vi "2nd_Order_ODE.vi"(2 "data":T1, 3 "t":dbl, 4 "x":dbl[](array[numeric])) -> (0 "error out":errorcluster, 1 "f(x,t)":dbl[](array[numeric]))   [LabVIEW 2012]
doc: "This template is the starting point for creating a function that is the right-hand-side of an ordinary differential equaltion to be passed to the ODE Solver.vi."
uses:
  <vilib>/gmath/NumericalOptimization/objective function data.ctl
  2nd_Order_TD.ctl
  <vilib>/gmath/NI_Gmath.lvlib
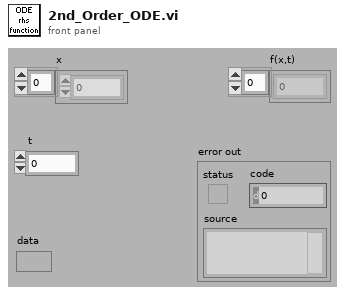
[diagram p1: front panel]
types:
  T1 = typedef "NI_Gmath.lvlib/objective function data.ctl" = variant
  T2 = typedef "2nd_Order_TD.ctl" = cluster{"omega_h":dbl, "zeta":dbl, "omega":dbl}
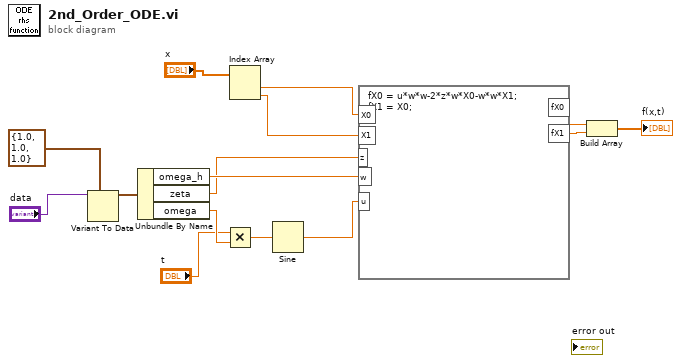
[diagram p0: block diagram]
diagram:
  n1 = Variant To Data(type=T2 {"omega_h"=1.0, "zeta"=1.0, "omega"=1.0} ("2nd Oder TD"), Variant="data") -> (data=w13:T2)  [unwired: 1 in, 1 out]
  n2 = Unbundle By Name(w13) -> ("omega_h"=w4:dbl, "zeta"=w3:dbl, "omega"=w12:dbl)
  n3 = Multiply(x="t", y=w12) -> (x*y=w10:dbl)
  n4 = Index Array(array="x") -> (element #1=w2:dbl, element #2=w1:dbl)  [unwired: 2 in]
  n5 = Sine(x=w10) -> (sin(x)=w5:dbl)
  n6 = formula code="fX0 = u*w*w-2*z*w*X0-w*w*X1;\nfX1 = X0;"("X0"=w2, "z"=w3, "w"=w4, "u"=w5, "X1"=w1) -> ("fX0"=w7:dbl, "fX1"=w8:dbl)
  n7 = Build Array(w7, w8) -> (→"f(x,t)":dbl[])
